vi "LaserOnOff.vi"() -> ()   [LabVIEW 2016]
uses:
  controls/Enum.ctl
  <vilib>/Utility/error.llb/Error Cluster From Error Code.vi
  <vilib>/rvi/errors/niLvFpgaAdjustHostInterfaceError.vi
  <vilib>/rvi/interface/nirviReadWriteControl/nirviReadWriteControl.xnode
  controls/FPGAVIreferenceTypeDefScanEngine.ctl
  FPGA Bitfiles/qnmController797_usbRIO_controllerFPGAmu.lvbitx
  NiFpgaLv.dll
panel:
  in  "ON/OFF":bool
  out "LASER":bool
  # "OFF"
  # "ON"
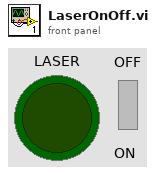
[diagram p1: front panel]
types:
  T1 = typedef "Enum.ctl" = enum16{"Init", "Read", "Write"}
  T2 = typedef "FPGAVIreferenceTypeDefScanEngine.ctl" = refnum<k20>
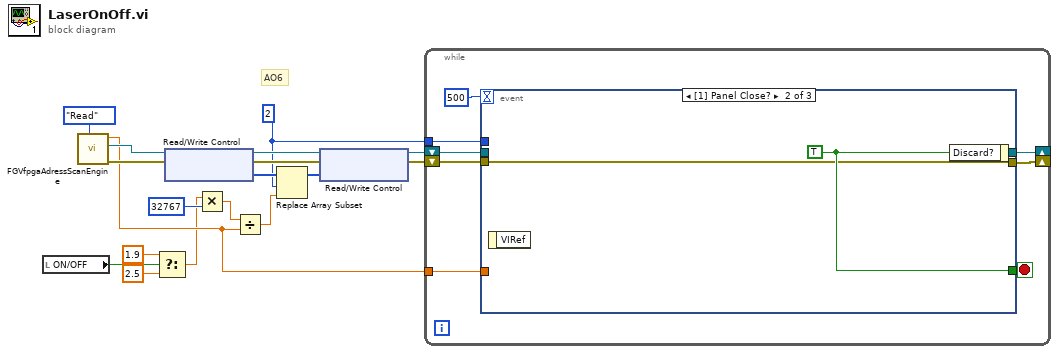
[diagram p0: block diagram]
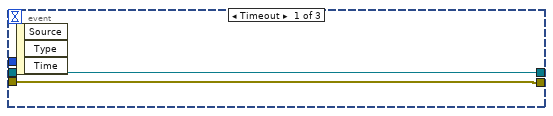
[diagram p2: hidden frame]
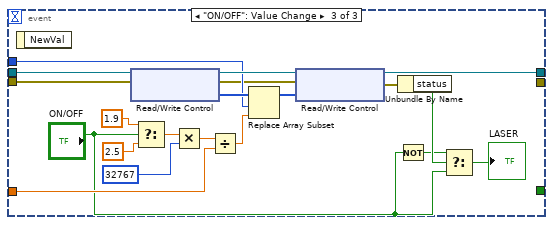
[diagram p3: hidden frame]
diagram:
  w8 = 2 ("index")
  # "AO6"
  n1 = local read "ON/OFF"() -> (w1:bool)
  n2 = call "FGVfpgaAdressScanEngine.vi"("Enum"=Enum."Read") -> ("error out"=w11:errorcluster, "FPGA.SEout"=w13:T2, "voltageRange(+/-)Out"=w5:dbl)  [unwired: 6 in, 2 out]
  n3 = Select(t=1.9, s=w1, f=2.5) -> (s? t:f=w2:dbl)
  n4 = xnode "Read/Write Control"("FPGA VI Reference In"=w13, "error in"=w11) -> ("FPGA VI Reference Out"=w10:T2, "error out"=w9:errorcluster, "aio.o.outputs"=w14:i16[])
  n5 = Multiply(x=w2, y=i16 32767) -> (x*y=w17:dbl)
  n6 = Divide(x=w17, y=w5) -> (x/y=w7:dbl)
  n7 = Replace Array Subset(array=w14, new element=w7, index=w8) -> (w15:i16[])
  n8 = xnode "Read/Write Control"("FPGA VI Reference In"=w10, "error in"=w9, "aio.o.outputs"=w15) -> ("FPGA VI Reference Out"=w12:T2, "error out"=w6:errorcluster)
  n9 = while {
    shift-right: [w24] -> _
    shift-left: w12 -> [w25]
    tunnel: w8 -> [w22]
    tunnel: w5 -> [w21]
    shift-right: [w19] -> _
    shift-left: w6 -> [w20]
    stop <- w23 stop-if-true
    n10 = event shown="[1] Panel Close?" {
      selector: _ -> [_ _ _]
      dyn-events: _ -> [_ _ _]
      timeout: 500 -> [_ _ _]
      tunnel: w25 -> [w28 _ w50]
      tunnel: [w28 _ w46] -> w24
      tunnel: [_ w30 _] -> w23
      tunnel: w22 -> [_ _ w42]
      tunnel: w21 -> [_ _ w41]
      tunnel: w20 -> [w27 w29 w40]
      tunnel: [w27 w29 _] -> w19
      event Timeout {
        n11 = event-data() -> ()  [unwired: 1 in, 3 out]
      }
      event Panel Close? {
        w30 = TRUE
        n12 = event-data() -> ()  [unwired: 1 in, 1 out]
        n13 = event-data("Discard?"=w30) -> ()  [unwired: 1 in, 1 out]
      }
      event "ON/OFF": Value Change {
        n14 = event-data() -> ()  [unwired: 1 in, 1 out]
        n15 = xnode "Read/Write Control"("FPGA VI Reference In"=w50, "error in"=w40) -> ("FPGA VI Reference Out"=w49:T2, "error out"=w39:errorcluster, "aio.o.outputs"=w48:i16[])
        n16 = Select(t=1.9, s="ON/OFF", f=2.5) -> (s? t:f=w38:dbl)
        n17 = Multiply(x=w38, y=i16 32767) -> (x*y=w44:dbl)
        n18 = Divide(x=w44, y=w41) -> (x/y=w43:dbl)
        n19 = Replace Array Subset(array=w48, new element=w43, index=w42) -> (w47:i16[])
        n20 = xnode "Read/Write Control"("FPGA VI Reference In"=w49, "error in"=w39, "aio.o.outputs"=w47) -> ("FPGA VI Reference Out"=w46:T2, "error out"=w35:errorcluster)
        n21 = Unbundle By Name(w35) -> ("status"=w34:bool)
        n22 = Not(x="ON/OFF") -> (.not. x?=w32:bool)
        n23 = Select(t=w32, s=w34, f="ON/OFF") -> (s? t:f=→"LASER":bool)
      }
    }
  }
